vi "Post_Process_Raw_data.vi"(0 "Select Plug Ins":bool, 2 "Post processed Results folder":path, 3 "No dialogs":bool, 5 "Save results to":T1(ring)=enum."Original Results Filenames with _PP", 9 "Per Block Plug Ins Extra":string[](array[string]), 11 "Selected files":path[](array[path]), 12 "Current Results filenames":path[](array[path]), 13 "Results Plotter Channel names":string[](array[string]), 14 "Results Plotter Data":string[][](array[string])) -> (4 "Stopped":bool, 15 "Post processed Results folder Out":path)   [LabVIEW 2016]
uses:
  Anemometry Sub Vis/Controls/File_Selector_Type.ctl
  Anemometry Sub Vis/Controls/Setup.ctl
  Anemometry Sub Vis/Controls/Post_Process.ctl
  Anemometry Sub Vis/Controls/Save_Data.ctl
  Anemometry Sub Vis/Globals/Meas_global.vi
  Anemometry Sub Vis/Data_plotting_vis/Results_plotter_Global.vi
  Anemometry Sub Vis/Globals/Plug_in_data_global.vi
  Anemometry Sub Vis/Globals/Dynamic_call_global.ph.vi
panel:
  out "Single Filename":string
  out "nFiles not found":i32
  out "Files not Found":path[](array[path])
  out "Checking":i32
  in  "Previous Choice":path
  in  "Search String":string
  in  "Proceed?":bool
  in  "Pause Mode":enum16{"Continuous Running", "After Each File"}(ring)
  in  "At Dialog Prompt Post Process":T2=enum."All files listed in selected file"
  out "Files Processed":i32(slide) scale=0.0..7.0
  in  "stop":bool
  out "Files To Process":path[](array[path])
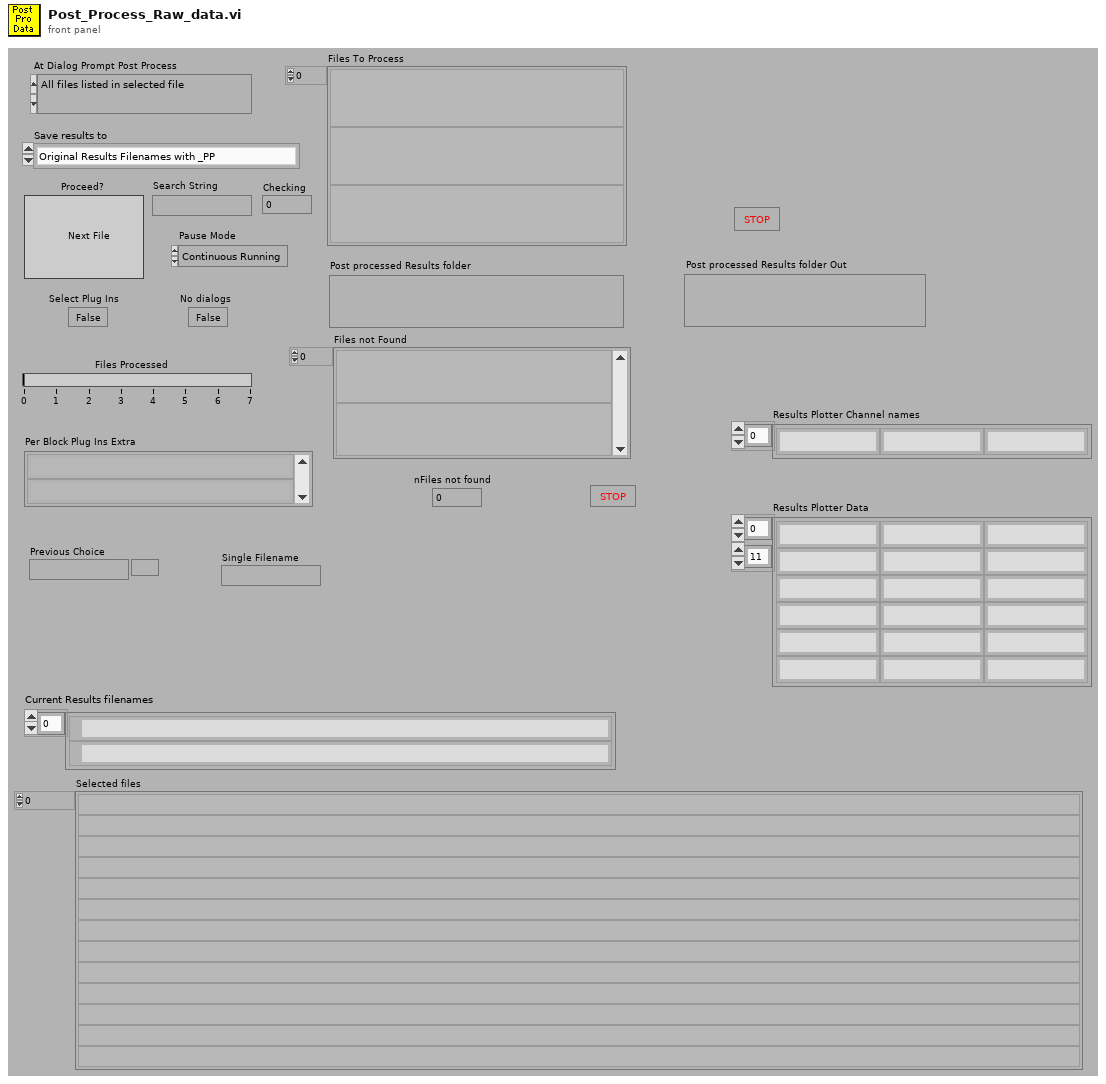
[diagram p1: front panel]
types:
  T1 = enum16{"A single file", "Original Results Filenames with _PP", "Current Results Filenames"}
  T2 = typedef "File_Selector_Type.ctl" = enum16{"The Selected File", "The Selected Folder", "Files containing the search string in the selected folder", "All files listed in selected file"}
  T3 = typedef "Setup.ctl" = enum16{"Run Program", "Show Setup", "Save Current Setup", "Setup Front Panel"}
  T4 = typedef "Save_Data.ctl" = enum16{"Save No Data", "Save Data"}
  T5 = typedef "Post_Process.ctl" = enum16{"Take New Data", "Post Process Raw Data File"}
  T6 = enum16{"Left Button", "Center Button", "Right Button", "Window Close"}
  T7 = typedef "Dispose_Channel.ctl" = enum16{"Always", "If Blank", "Never"}
  T8 = typedef "Multi_Run_Status.ctl" = enum16{"Continue", "Jump to Next Point", "Jump to Next Row", "Jump To Fall Back", "Terminate Run"}
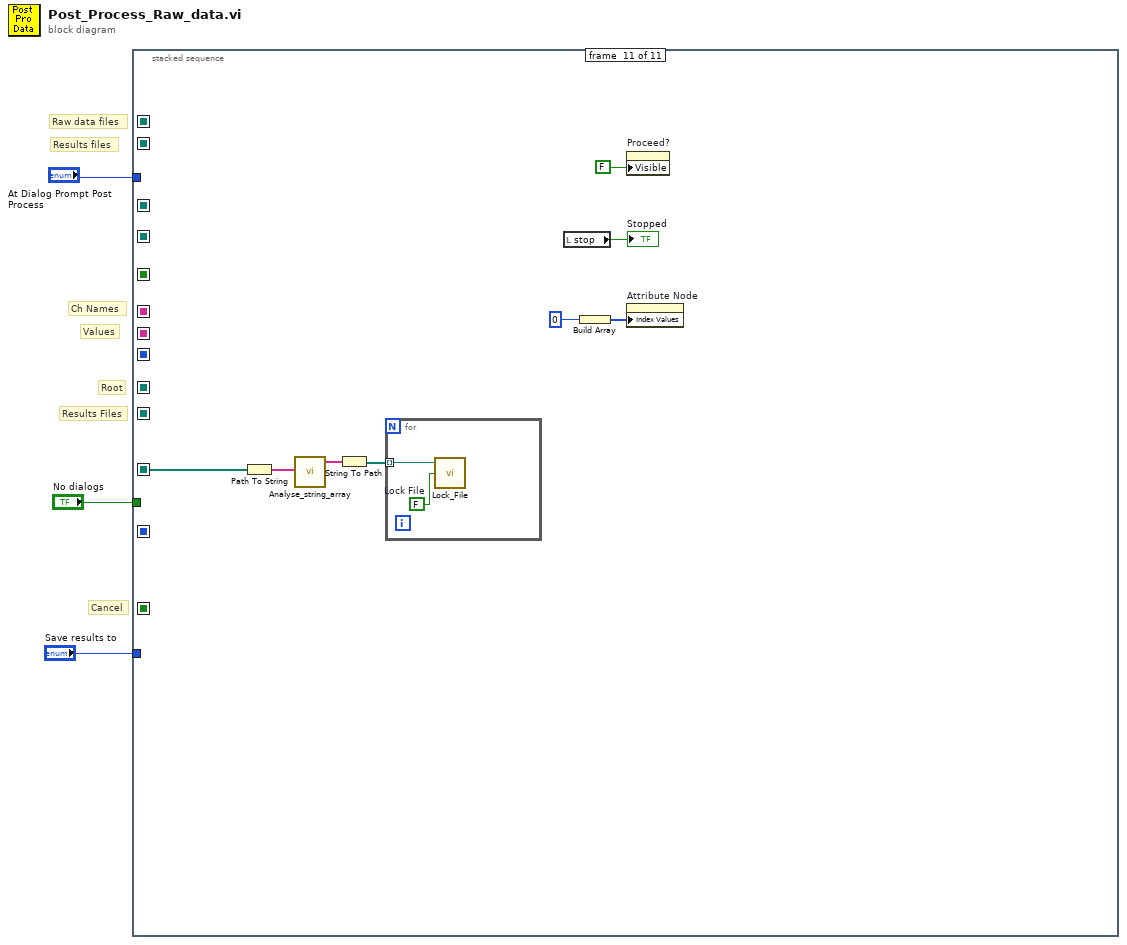
[diagram p0: block diagram]
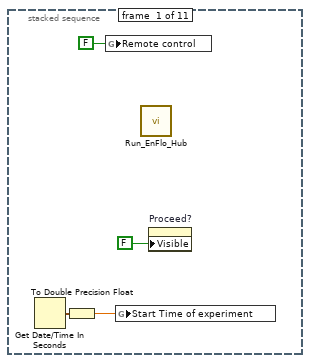
[diagram p2: hidden frame]
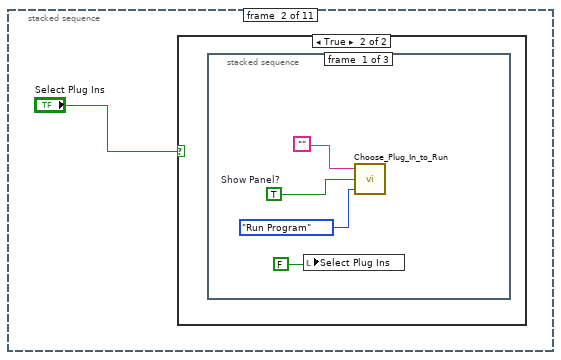
[diagram p3: hidden frame]
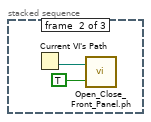
[diagram p5: hidden frame]
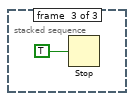
[diagram p6: hidden frame]
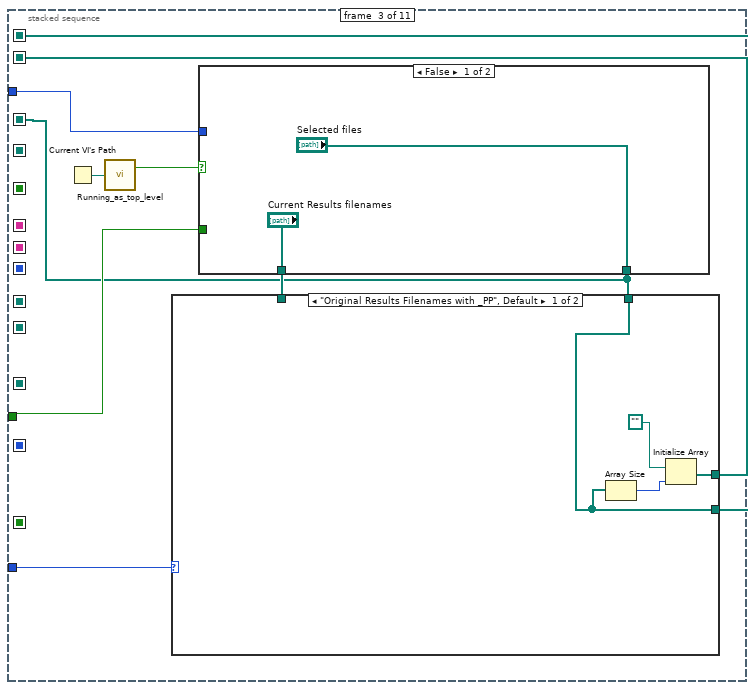
[diagram p7: hidden frame]
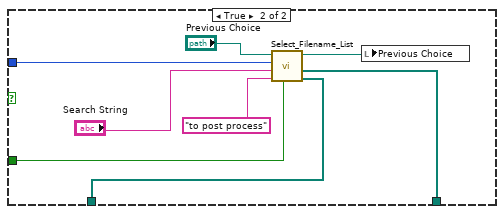
[diagram p9: hidden frame]
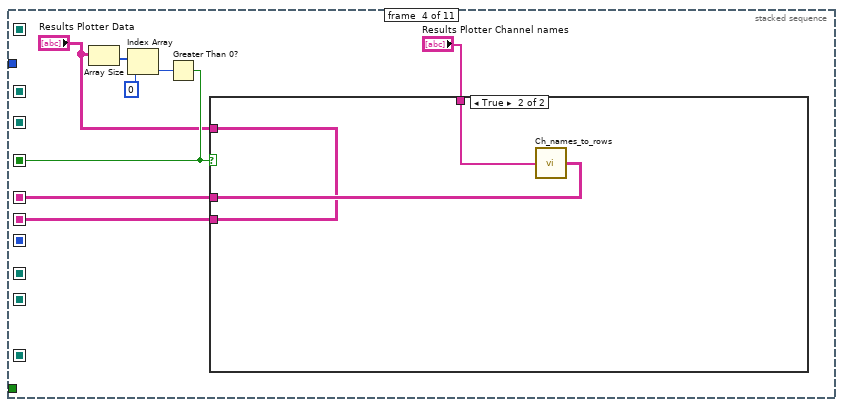
[diagram p10: hidden frame]
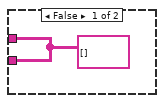
[diagram p11: hidden frame]
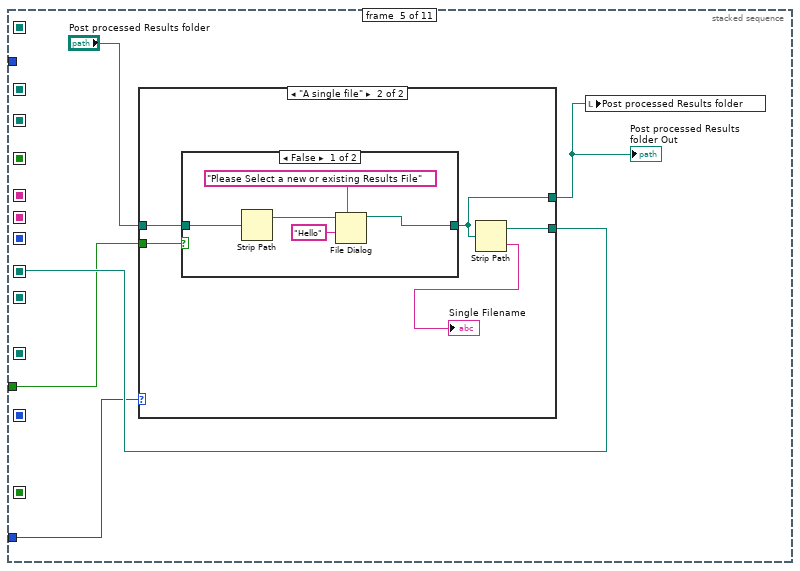
[diagram p12: hidden frame]
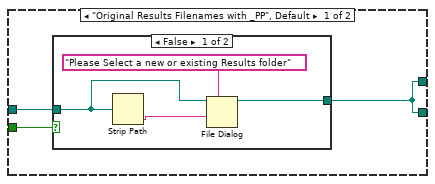
[diagram p13: hidden frame]
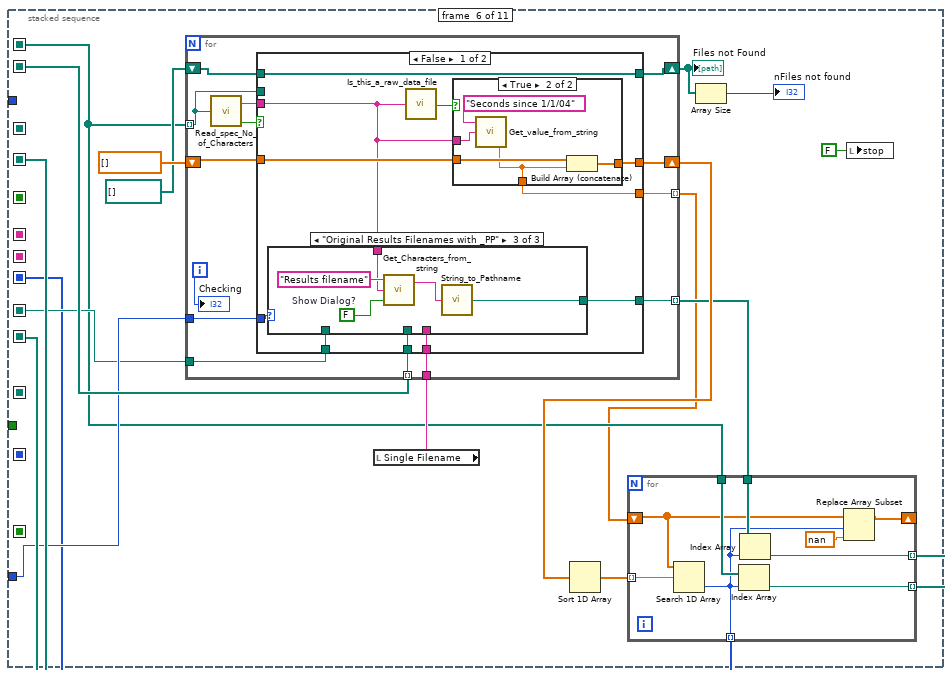
[diagram p16: hidden frame]
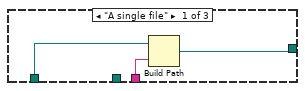
[diagram p17: hidden frame]
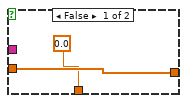
[diagram p19: hidden frame]
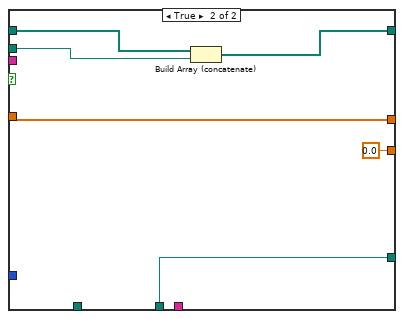
[diagram p20: hidden frame]
diagram:
  # "Values"
  # "Ch Names"
  # "Cancel"
  # "Results files"
  # "Raw data files"
  # "Root"
  # "Results Files"
  n1 = stacked-sequence {
    seq-local: [_ _ _ _ _ w90 _ _ _ _ _] -> [_ _ _ _ _ _ _ _ w222 w235 _]
    seq-local: [_ _ _ _ _ _ _ _ w227 _ _] -> [_ _ _ _ _ _ _ _ _ w234 _]
    seq-local: [_ _ w18 _ _ _ _ _ _ _ _] -> [_ _ _ _ _ w79 _ _ _ _ _]
    seq-local: [_ _ _ _ w57 _ _ _ _ _ _] -> [_ _ _ _ _ w82 w151 _ _ _ _]
    seq-local: [_ _ _ _ _ w88 _ _ _ _ _] -> [_ _ _ _ _ _ w154 _ _ _ _]
    seq-local: [_ _ _ _ _ _ w150 _ _ _ _] -> [_ _ _ _ _ _ _ w194 _ w233 w343]
    seq-local: [_ _ w19 _ _ _ _ _ _ _ _] -> [_ _ _ _ _ w84 _ _ _ _ _]
    seq-local: [_ _ _ w48 _ _ _ _ _ _ _] -> [_ _ _ _ _ _ _ _ _ w232 _]
    seq-local: [_ _ _ w47 _ _ _ _ _ _ _] -> [_ _ _ _ _ _ _ _ _ w229 _]
    seq-local: [_ _ _ w43 _ _ _ _ _ _ _] -> [_ _ _ _ _ _ _ _ _ w231 _]
    seq-local: [_ _ _ _ _ w80 _ _ _ _ _] -> [_ _ _ _ _ _ _ _ _ w230 _]
    seq-local: [_ _ w16 _ _ _ _ _ _ _ _] -> [_ _ _ _ _ _ _ _ _ _ _]
    seq-local: [_ _ _ _ _ _ _ w196 _ _ _] -> [_ _ _ _ _ _ _ _ _ w228 _]
    tunnel: "At Dialog Prompt Post Process" -> [_ _ w24 _ _ _ _ _ _ _ _]
    tunnel: "No dialogs" -> [_ _ w23 _ w55 _ _ w197 _ _ _]
    tunnel: "Save results to" -> [_ _ w17 _ w54 w83 w153 _ _ _ _]
    frame #0 {
      n2 = Get Date/Time In Seconds() -> (seconds since 1Jan1904=w4:timestamp)
      n3 = To Double Precision Float(number=w4) -> (double precision float=w5:dbl)
      n4 = global write "Meas_global.vi" "Remote control"(FALSE ("Remote control")) -> ()
      n5 = global write "Meas_global.vi" "Start Time of experiment"(w5) -> ()
      n6 = call "Run_EnFlo_Hub.vi"() -> ()  [unwired: 1 in, 7 out]
      n7 = property on="Proceed?" class="Bool"("Visible"=FALSE ("Write Attribute")) -> ()  [unwired: 2 in, 2 out]
    }
    frame #1 {
      n8 = case shown="True" "Select Plug Ins" {
        frame False {
        }
        frame True {
          n9 = stacked-sequence {
            frame #0 {
              w12 = TRUE  # Show Panel?
              n10 = local write "Select Plug Ins"(FALSE ("Select Local ADAM Channels")) -> ()
              n11 = call "Choose_Plug_In_to_Run.vi"("setup"=Setup."Run Program", "Show Panel?"=w12, "Setup String In"="") -> ()  [unwired: 2 out]
            }
            frame #1 {
              n12 = Current VI's Path() -> (path=w14:path)
              n13 = call "Open_Close_Front_Panel.ph.vi"("Front Panel Window:Open"=TRUE, "VI path"=w14) -> ()  [unwired: 2 out]
            }
            frame #2 {
              n14 = Stop(stop? (T)=TRUE) -> ()
            }
          }
        }
      }
    }
    frame #2 {
      n15 = Current VI's Path() -> (path=w22:path)
      n16 = call "Running_as_top_level.vi"("Vi path name"=w22) -> ("Top Level"=w21:bool)  [unwired: 1 out]
      n17 = case shown="False" w21 {
        tunnel: w24 -> [_ w40]
        tunnel: w23 -> [_ w35]
        tunnel: ["Selected files" w34] -> w16
        tunnel: ["Current Results filenames" w33] -> w20
        frame False {
        }
        frame True {
          n18 = call "Select_Filename_List.vi"("No dialogs"=w35, "File Type"="to post process", "Search String"="Search String", "At Dialog Prompt Post Process"=w40, "Previous Choice"="Previous Choice") -> ("Current Results filenames"=w33:path[], "Selected files"=w34:path[], "Choosen path"=w36:path)  [unwired: 1 out]
          n19 = local write "Previous Choice"(w36) -> ()
        }
      }
      n20 = case shown="\"Original Results Filenames with _PP\", Default" w17 {
        tunnel: w16 -> [w25 w29]
        tunnel: w20 -> [_ w30]
        tunnel: [w27 w30] -> w19
        tunnel: [w25 w29] -> w18
        frame "Original Results Filenames with _PP", Default {
          n21 = Array Size(array=w25) -> (size(s)=w28:i32)
          n22 = Initialize Array(path "", w28) -> (w27:path[])
        }
        frame "Current Results Filenames" {
        }
      }
    }
    frame #3 {
      n23 = Array Size(array="Results Plotter Data") -> (size(s)=w46:i32[])
      n24 = Index Array(array=w46, index=0) -> (element=w44:i32)
      n25 = Greater Than 0?(x=w44) -> (x > 0?=w43:bool)
      n26 = case shown="True" w43 {
        tunnel: [w49 w52] -> w48
        tunnel: [w49 w50] -> w47
        tunnel: "Results Plotter Data" -> [_ w50]
        tunnel: "Results Plotter Channel names" -> [_ w51]
        frame False {
          w49 = string[][] [] ("3 Row names")
        }
        frame True {
          n27 = call "Ch_names_to_rows.vi"("Channel Names"=w51) -> ("3 Row names"=w52:string[][])
        }
      }
    }
    frame #4 {
      n28 = case shown="\"A single file\"" w54 {
        tunnel: [w58 w67] -> w57
        tunnel: "Post processed Results folder" -> [w60 w70]
        tunnel: w55 -> [w59 w69]
        tunnel: [w58 w68] -> w53
        frame "Original Results Filenames with _PP", Default {
          n29 = case shown="False" w59 {
            tunnel: [w64 w65] -> w58
            tunnel: w60 -> [w61 w65]
            frame False {
              n30 = Strip Path(path=w61) -> (name=w62:string)  [unwired: 1 out]
              n31 = File Dialog(7:"Please Select a new or existing Results folder" ("prompt"), 9:w62, 11:w61) -> (3:w64:path)  [unwired: 1 in, 6 out]
            }
            frame True {
            }
          }
        }
        frame "A single file" {
          n32 = case shown="False" w69 {
            tunnel: w70 -> [w74 w76]
            tunnel: [w73 w76] -> w68
            frame False {
              n33 = Strip Path(path=w74) -> (stripped path=w72:path)  [unwired: 1 out]
              n34 = File Dialog(7:"Please Select a new or existing Results File" ("prompt"), 9:"Hello" ("default name"), 11:w72) -> (3:w73:path)  [unwired: 1 in, 6 out]
            }
            frame True {
            }
          }
          n35 = Strip Path(path=w68) -> (stripped path=w67:path, name=→"Single Filename":string)
        }
      }
      "Post processed Results folder Out" <- w53
      n36 = local write "Post processed Results folder"(w53) -> ()
    }
    frame #5 {
      n37 = local read "Single Filename"() -> (w81:string)
      n38 = for {
        tunnel: w79 -> [w111] mode=indexing
        shift-right: [w115] -> w93
        shift-left: dbl[] [] -> [w116]
        shift-right: [w112] -> w86
        shift-left: path[] [] -> [w113]
        tunnel: w84 -> [w108] mode=indexing
        tunnel: w83 -> [w107]
        tunnel: w82 -> [w106]
        tunnel: w81 -> [w105]
        tunnel: [w104] -> w78 mode=indexing
        tunnel: [w103] -> w77 mode=indexing
        i -> [w114]
        n39 = call "Read_spec_No_of_Characters.vi"("Filename"=w111) -> ("character string"=w110:string, "Error?"=w109:bool)
        n40 = case shown="False" w109 {
          tunnel: w116 -> [w127 w149]
          tunnel: [w126 w149] -> w115
          tunnel: w111 -> [_ w147]
          tunnel: w113 -> [w124 w148]
          tunnel: [w124 w146] -> w112
          tunnel: w110 -> [w123 _]
          tunnel: w108 -> [w121 w145]
          tunnel: w107 -> [w122 _]
          tunnel: w106 -> [w120 _]
          tunnel: w105 -> [w119 _]
          tunnel: [w118 w145] -> w104
          tunnel: [w117 0.0 ("Value")] -> w103
          frame False {
            n41 = case shown="\"Original Results Filenames with _PP\"" w122 {
              tunnel: [w130 w131 w134] -> w118
              tunnel: w123 -> [_ _ w132]
              tunnel: w121 -> [_ w131 _]
              tunnel: w120 -> [w129 _ _]
              tunnel: w119 -> [w128 _ _]
              frame "A single file" {
                n42 = Build Path(base path=w129, name or relative path=w128) -> (appended path=w130:path)
              }
              frame "Current Results Filenames" {
              }
              frame "Original Results Filenames with _PP" {
                w135 = FALSE  # Show Dialog?
                n43 = call "Get_Characters_from_string.vi"("Show Dialog?"=w135, "Input string"=w132, "Variable name"="Results filename") -> ("Value"=w133:string)  [unwired: 1 out]
                n44 = call "String_to_Pathname.vi"("Input String"=w133) -> ("path"=w134:path)
              }
            }
            n45 = call "Is_this_a_raw_data_file.vi"("character string"=w123) -> ("Raw Dat File?"=w125:bool)  [unwired: 2 out]
            n46 = case shown="True" w125 {
              tunnel: w127 -> [w138 w140]
              tunnel: [w138 w143] -> w126
              tunnel: w123 -> [_ w141]
              tunnel: [0.0 ("Value") w139] -> w117
              frame False {
              }
              frame True {
                n47 = call "Get_value_from_string.vi"("Input string"=w141, "Variable name"="Seconds since 1/1/04") -> ("Value"=w139:dbl)  [unwired: 1 in, 1 out]
                n48 = Build Array (concatenate)(w140, w139) -> (w143:dbl[])
              }
            }
          }
          frame True {
            n49 = Build Array (concatenate)(w148, w147) -> (w146:path[])
          }
        }
        "Checking" <- w114
      }
      "Files not Found" <- w86
      n50 = Sort 1D Array(array=w93) -> (sorted array=w92:dbl[])
      n51 = for {
        tunnel: w92 -> [w102] mode=indexing
        tunnel: w79 -> [w101]
        tunnel: [w100] -> w90 mode=indexing
        tunnel: w78 -> [w99]
        tunnel: [w98] -> w88 mode=indexing
        tunnel: [w96] -> w80 mode=indexing
        shift-right: [w97] -> _
        shift-left: w77 -> [w94]
        n52 = Search 1D Array(1D array=w94, element=w102) -> (index of element=w96:i32)  [unwired: 1 out]
        n53 = Index Array(array=w101, index=w96) -> (element=w100:path)
        n54 = Index Array(array=w99, index=w96) -> (element=w98:path)
        n55 = Replace Array Subset(array=w94, new element=nan ("new element/subarray"), index=w96) -> (w97:dbl[])
      }
      n56 = Array Size(array=w86) -> (size(s)=→"nFiles not found":i32)
      n57 = local write "stop"(FALSE ("stop")) -> ()
    }
    frame #6 {
      n58 = case shown="\"Original Results Filenames with _PP\"" w153 {
        tunnel: [FALSE TRUE] -> w152
        tunnel: w153 -> [_ _]
        frame "A single file", Default {
        }
        frame "Original Results Filenames with _PP" {
        }
      }
      n59 = for {
        tunnel: w154 -> [w188] mode=indexing
        tunnel: w152 -> [w160]
        tunnel: w151 -> [w159]
        tunnel: [w157] -> w150 mode=indexing
        w173 = "_" ("Replace with")
        n60 = Strip Path(path=w188) -> (name=w161:string)  [unwired: 1 out]
        n61 = Concatenate Strings("[" ("Substring"), ":", "/", "\\\\", "|", "?", ">", "<", "*", "\"", "]" ("Substring")) -> (w176:string)
        n62 = call <vilib>:"Trim Whitespace.vi"("string"=w161) -> ("trimmed string"=w175:string)  [unwired: 1 in]
        n63 = call "Add_filename_suffix.vi"("Filename"=w175) -> ("Original Suffix"=w165:string, "Base name"=w174:string)  [unwired: 1 in, 2 out]
        n64 = call "Replace_Character.vi"("Replace with"=w173, "Input String"=w174, "Search For"=w176) -> ("Output string"=w169:string)  [unwired: 1 out]
        n65 = call "Replace_Character.vi"("Replace with"="_", "Input String"=w169, "Search For"=" ") -> ("Output string"=w170:string)  [unwired: 1 out]
        n66 = case shown="False" w160 {
          tunnel: [w189 w191] -> w172
          tunnel: w170 -> [w189 w190]
          frame False {
          }
          frame True {
            n67 = Concatenate Strings(w190, "_pp" ("Substring")) -> (w191:string)
          }
        }
        n68 = Empty String/Path?(string/path=w165) -> (empty?=w166:bool)
        n69 = Select(t=".xls", s=w166, f=w165) -> (s? t:f=w164:string)
        n70 = call "Replace_Character.vi"("Replace with"=w173, "Input String"=w172, "Search For"="__") -> ("Output string"=w163:string)  [unwired: 1 out]
        n71 = Concatenate Strings(w163, w164) -> (w158:string)
        n72 = Build Path(base path=w159, name or relative path=w158) -> (appended path=w157:path)
      }
    }
    frame #7 {
      n73 = Path To String(path=w194) -> (string=w195:string[])
      n74 = call "Analyse_string_array.vi"("String array"=w195) -> ("Unique strings"=w193:string[])  [unwired: 2 out]
      n75 = case shown="False" w197 {
        tunnel: [w199 FALSE ("stop? (T)")] -> w196
        tunnel: w193 -> [w198 w218]
        frame False {
          n76 = for {
            tunnel: w198 -> [w202] mode=indexing
            tunnel: [w201] -> w199
            stop <- w201 stop-if-true
            n77 = String To Path(string=w202) -> (path=w200:path)
            n78 = call "Create_directory_path.vi"("Path name"=w200) -> ()  [unwired: 2 in, 2 out]
            n79 = call "Does_file_exist_(simple).vi"("Pathname"=w200) -> ("exists?"=w203:bool)
            n80 = case shown="True" w203 {
              tunnel: w200 -> [_ w208]
              tunnel: [FALSE ("stop? (T)") w207] -> w201
              frame False {
              }
              frame True {
                n81 = Format Into String(format string="%s\nAlready exists. ", w208) -> (resulting string=w211:string)  [unwired: 2 in, 1 out]
                n82 = call <vilib>:"Three Button Dialog.vi"("Allow user to close window? (TRUE)"=FALSE, "Center Button Text (\"No\")"="Append" ("Center Button Text (\"No\")"), "Left Button Text (\"Yes\")"="Overwrite" ("Left Button Text (\"Yes\")"), "message"=w211) -> ("Which Button?"=w209:T6)  [unwired: 7 in]
                n83 = case shown="\"Center Button\"" w209 {
                  tunnel: w208 -> [w214 _ _ _]
                  tunnel: [FALSE ("stop? (T)") FALSE ("stop? (T)") TRUE ("stop? (T)") FALSE ("stop? (T)")] -> w207
                  frame "Left Button" {
                    n84 = Delete(path (use dialog)=w214) -> ()  [unwired: 4 in, 3 out]
                  }
                  frame "Center Button" {
                  }
                  frame "Right Button" {
                  }
                  frame "Window Close" {
                  }
                }
              }
            }
          }
        }
        frame True {
          n85 = for {
            tunnel: w218 -> [w221] mode=indexing
            n86 = String To Path(string=w221) -> (path=w220:path)
            n87 = call "Create_directory_path.vi"("Path name"=w220) -> ()  [unwired: 2 in, 2 out]
          }
        }
      }
    }
    frame #8 {
      w223 = 0 ("Files Processed")
      n88 = Array Size(array=w222) -> (size(s)=w227:i32)
      n89 = Array Size(array=w222) -> (size(s)=w225:i32)
      n90 = property on="Files Processed" class="Slide (strict)"("Scale.Range:Minimum"=0.0 ("Write Attribute"), "Scale.Range:Maximum"=w225) -> ()  [unwired: 2 in, 2 out]
      n91 = Build Array(w223) -> (w224:i32[])
      n92 = property on="Attribute Node" class="Arr (strict)"("Index Values"=w224) -> ()  [unwired: 2 in, 2 out]
      n93 = local write "Files Processed"(w223) -> ()
      "Files To Process" <- w222
    }
    frame #9 {
      n94 = case shown="False" w228 {
        tunnel: w235 -> [w242 _]
        tunnel: w234 -> [w241 _]
        tunnel: w233 -> [w240 _]
        tunnel: w232 -> [w239 _]
        tunnel: w231 -> [w238 _]
        tunnel: w230 -> [w237 _]
        tunnel: w229 -> [w236 _]
        frame False {
          n95 = while {
            tunnel: w240 -> [w247] mode=indexing
            tunnel: w241 -> [w250]
            tunnel: w242 -> [w251] mode=indexing
            tunnel: w239 -> [w246]
            tunnel: w237 -> [w243] mode=indexing
            tunnel: w238 -> [w245]
            tunnel: w236 -> [w244]
            i -> [w249]
            stop <- w248 continue-if-true
            n96 = stacked-sequence {
              seq-local: [_ _ _ w314 _ _] -> [_ _ _ _ w318 _]
              seq-local: [w255 _ _ _ _ _] -> [_ w271 _ _ _ _]
              seq-local: [w252 _ _ _ _ _] -> [_ w270 _ _ _ _]
              tunnel: w247 -> [_ _ _ w316 _ _]
              tunnel: w251 -> [_ _ _ w315 _ _]
              tunnel: w250 -> [_ _ _ _ w320 _]
              tunnel: w249 -> [_ _ _ _ w319 w339]
              tunnel: [_ _ _ _ w317 _] -> w248
              tunnel: w246 -> [_ w275 _ _ _ _]
              tunnel: w245 -> [_ w274 _ _ _ _]
              tunnel: w244 -> [w257 _ _ _ _ _]
              tunnel: w243 -> [w254 _ _ _ _ _]
              frame #0 {
                n97 = Index Array(array=w257, index (row)=w254) -> (element=w253:string[])  [unwired: 1 in]
                n98 = Build Array(w253) -> (w252:string[][])
                n99 = global read "Results_plotter_Global.vi" "Dispose"() -> (w256:T7[])
                n100 = for {
                  tunnel: w256 -> [w261] mode=indexing
                  tunnel: [w258] -> w255 mode=indexing if=w260
                  tunnel: w252 -> [w259]
                  i -> [w258]
                  n101 = case shown="\"If Blank\"" w261 {
                    tunnel: [FALSE TRUE w264] -> w260
                    tunnel: w259 -> [_ _ w269]
                    tunnel: w258 -> [_ _ w268]
                    frame "Always" {
                    }
                    frame "Never" {
                    }
                    frame "If Blank" {
                      n102 = Index Array(array=w269, index (col)=w268) -> (element=w267:string[])  [unwired: 1 in]
                      n103 = Concatenate Strings(w267) -> (w266:string)
                      n104 = Empty String/Path?(string/path=w266) -> (empty?=w265:bool)
                      n105 = Not(x=w265) -> (.not. x?=w264:bool)
                    }
                  }
                }
              }
              frame #1 {
                n106 = case shown="True" w274 {
                  tunnel: w275 -> [_ w283]
                  tunnel: w270 -> [_ w281]
                  tunnel: [w276 w278] -> w273
                  tunnel: [w276 w281] -> w272
                  tunnel: w271 -> [_ w282]
                  frame False {
                    w276 = string[][] [] ("3 Row names")
                  }
                  frame True {
                    n107 = global read "Results_plotter_Global.vi" "Precision"() -> (w277:string[])
                    n108 = for {
                      tunnel: w282 -> [w287]
                      tunnel: w281 -> [w286] mode=indexing
                      tunnel: w277 -> [w285]
                      tunnel: [w284] -> w280 mode=indexing
                      n109 = for {
                        tunnel: w287 -> [w297] mode=indexing
                        tunnel: w286 -> [w299]
                        tunnel: w285 -> [w298]
                        tunnel: [w291] -> w284 mode=indexing
                        n110 = Index Array(array=w299, index=w297) -> (element=w290:string)
                        n111 = Index Array(array=w298, index=w297) -> (element=w289:string)
                        n112 = Fract/Exp String To Number(string=w290) -> (offset past number=w295:i32, number=w292:dbl)  [unwired: 3 out]
                        n113 = String Length(string=w290) -> (length=w296:i32)
                        n114 = Equal?(x=w296, y=w295) -> (x = y?=w293:bool)
                        n115 = Empty String/Path?(string/path=w290) -> (empty?=w294:bool)
                        n116 = Compound Arithmetic op=AND(invert w294, w293) -> (w288:bool)
                        n117 = case shown="False" w288 {
                          tunnel: w289 -> [_ w302]
                          tunnel: w292 -> [_ w303]
                          tunnel: [w300 w301] -> w291
                          tunnel: w290 -> [w300 _]
                          frame False {
                          }
                          frame True {
                            n118 = call "Number_2_string.vi"("precision"=w302, "number"=w303) -> ("String"=w301:string)
                          }
                        }
                      }
                    }
                    n119 = for {
                      tunnel: w282 -> [w305]
                      tunnel: w283 -> [w306] mode=indexing
                      tunnel: [w304] -> w279 mode=indexing
                      n120 = for {
                        tunnel: w305 -> [w309] mode=indexing
                        tunnel: w306 -> [w308]
                        tunnel: [w307] -> w304 mode=indexing
                        n121 = Index Array(array=w308, index=w309) -> (element=w307:string)
                      }
                    }
                    n122 = Build Array (concatenate)(w279, w280) -> (w278:string[][])
                  }
                }
                n123 = global write "Plug_in_data_global.vi" "Results File Plotter Rows"(w272) -> ()
                n124 = global write "Plug_in_data_global.vi" "Templated Results header"(w273) -> ()
              }
              frame #2 {
                n125 = global write "Dynamic_call_global.ph.vi" "Per Block Plug Ins Extra"("Per Block Plug Ins Extra") -> ()
              }
              frame #3 {
                n126 = call "Measurement.vi"("setup"=Setup."Run Program", "Post Process"=Post_Process."Post Process Raw Data File", "File"=Save_Data."Save Data", "Results file"=w316, "Raw data file"=w315) -> ("Status Out"=w314:T8)  [unwired: 2 in, 12 out]
              }
              frame #4 {
                n127 = Increment(x=w319) -> (x+1=w322:i32)
                n128 = Less?(x=w322, y=w320) -> (x < y?=w321:bool)
                n129 = while {
                  tunnel: [w329] -> w317
                  tunnel: w318 -> [w330]
                  tunnel: w321 -> [w324]
                  stop <- w327 continue-if-true
                  n130 = case shown="\"After Each File\"" "Pause Mode" {
                    tunnel: [TRUE "Proceed?"] -> w326
                    frame "Continuous Running" {
                    }
                    frame "After Each File" {
                      w333 = TRUE ("Blinking")
                      n131 = Wait (ms)(milliseconds to wait=u32 100 ("f")) -> ()  [unwired: 1 out]
                      n132 = property on="Proceed?" class="Bool"("Visible"=w333, "Key Focus"=w333, "Blinking"=w333) -> ()  [unwired: 2 in, 2 out]
                    }
                  }
                  n133 = Compound Arithmetic op=AND(invert w326, invert "stop", w324) -> (w327:bool)
                  n134 = Compound Arithmetic op=AND(w326, invert "stop", w324) -> (w323:bool)
                  n135 = case shown="\"Continue\", Default" w330 {
                    tunnel: [w335 FALSE] -> w329
                    tunnel: w323 -> [w335 _]
                    frame "Continue", Default {
                    }
                    frame "Terminate Run" {
                    }
                  }
                }
              }
              frame #5 {
                w337 = string[][] [] ("Results File Plotter Rows")
                n136 = Increment(x=w339) -> (x+1=w338:i32)
                "Files Processed" <- w338
                n137 = global write "Plug_in_data_global.vi" "Templated Results header"(w337) -> ()
                n138 = global write "Plug_in_data_global.vi" "Results File Plotter Rows"(w337) -> ()
                n139 = Build Array(w338) -> (w340:i32[])
                n140 = property on="Attribute Node" class="Arr (strict)"("Index Values"=w340) -> ()  [unwired: 2 in, 2 out]
              }
            }
          }
        }
        frame True {
        }
      }
    }
    frame #10 {
      n141 = Path To String(path=w343) -> (string=w345:string[])
      n142 = call "Analyse_string_array.vi"("String array"=w345) -> ("Unique strings"=w344:string[])  [unwired: 2 out]
      n143 = String To Path(string=w344) -> (path=w342:path[])
      n144 = for {
        tunnel: w342 -> [w349] mode=indexing
        w350 = FALSE  # Lock File
        n145 = call "Lock_File.vi"("Lock File"=w350, "path"=w349) -> ()  [unwired: 1 in, 3 out]
      }
      n146 = local read "stop"() -> (→"Stopped":bool)
      n147 = Build Array(0) -> (w347:i32[])
      n148 = property on="Proceed?" class="Bool"("Visible"=FALSE ("Write Attribute")) -> ()  [unwired: 2 in, 2 out]
      n149 = property on="Attribute Node" class="Arr (strict)"("Index Values"=w347) -> ()  [unwired: 2 in, 2 out]
    }
  }
